vi "DataLog List Tag Logs.vi"(7 "database path":path, 11 "error in (no error)":errorcluster) -> (8 "tag info list":T1[](array[typedef]) {"logging parameters" format="%.2e"; "precision" items=["0", "1", "2", "3", "4", "5", "6", "7", "8", "9", "10", "11", "12", "13", "14", "15", "16", "17"]; "limit delay" format="%.2e"; "deadband" format="%.2e"}, 15 "error out":errorcluster)   [LabVIEW 2012]
doc: "List the tag log directories in the data log base path as well as any meta tag log directories contained in these. The validity of the logs will be verified and the tag infos will be loaded and returned in an array."
uses:
  typedefs/clusters/t_DataLog Tag Config.ctl
  typedefs/t_DataLog Temporal Types.ctl
  typedefs/t_DataLog Value Types.ctl
  typedefs/t_DataLog Numerical Format.ctl
  typedefs/t_DataLog Logging Algorithms.ctl
  typedefs/et_DataLog Meta Tag Specifier.ctl
  glb_DataLog MCVD.vi
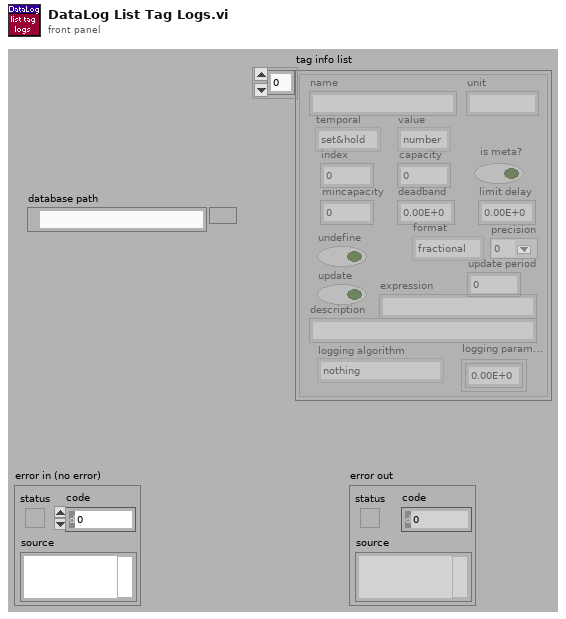
[diagram p1: front panel]
types:
  T1 = typedef "t_DataLog Tag Config.ctl" = cluster{"name":string, "unit":string, "temporal":T2, "value":T3, "index":i32, "capacity":i32, "is meta?":bool, "mincapacity":i32, "deadband":dbl, "limit delay":dbl, "format":T4, "precision":u8, "undefine":bool, "update":bool, "update period":u16, "expression":string, "description":string, "logging algorithm":T5, "logging parameters":dbl[]}
  T2 = typedef "t_DataLog Temporal Types.ctl" = enum16{"set&hold", "sample", "event"}
  T3 = typedef "t_DataLog Value Types.ctl" = enum16{"number", "string"}
  T4 = typedef "t_DataLog Numerical Format.ctl" = enum8{"fractional", "exponential", "engineering"}
  T5 = typedef "t_DataLog Logging Algorithms.ctl" = enum16{"nothing", "changes", "everything", "every Nth", "time threshold", "value threshold + prior", "t or v threshold", "t or v threshold + prior"}
  T6 = typedef "et_DataLog Meta Tag Specifier.ctl" = enum32{"warn_lo", "warn_hi", "A_lo", "A_hi", "B_lo", "B_hi", "C_lo", "C_hi", "D_lo", "D_hi", "E_lo", "E_hi", "F_lo", "F_hi", "G_lo", "G_hi", "H_lo", "H_hi", "I_lo", "I_hi", "J_lo", "J_hi", "K_lo", "K_hi", "L_lo", "L_hi", "M_lo", "M_hi", "N_lo", "N_hi", "min", "max", "not a meta"}
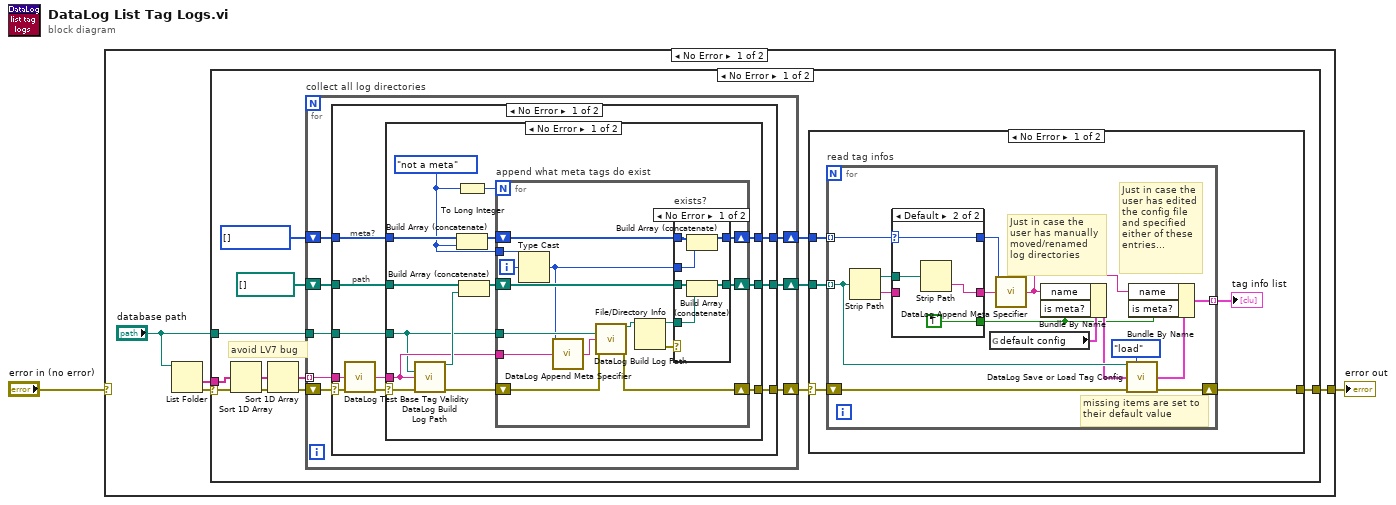
[diagram p0: block diagram]
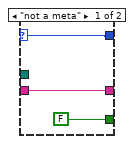
[diagram p2: hidden frame]
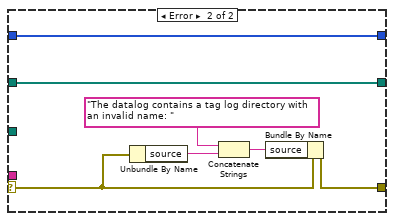
[diagram p5: hidden frame]
diagram:
  n1 = case shown="No Error" "error in (no error)" {
    selector: "error in (no error)" -> [_ w112]
    tunnel: [w6 w112] -> w2
    frame No Error {
      n2 = List Folder(path="database path") -> (folder names=w4:string[], error out=w5:errorcluster)  [unwired: 3 in, 2 out]
      n3 = case shown="No Error" w5 {
        selector: w5 -> [w16 w111]
        tunnel: [w14 w111] -> w6
        tunnel: w4 -> [w7 _]
        tunnel: "database path" -> [w10 _]
        frame No Error {
          w12 = T6[] [] items=["warn_lo", "warn_hi", "A_lo", "A_hi", "B_lo", "B_hi", "C_lo", "C_hi", "D_lo", "D_hi", "E_lo", "E_hi", "F_lo", "F_hi", "G_lo", "G_hi", "H_lo", "H_hi", "I_lo", "I_hi", "J_lo", "J_hi", "K_lo", "K_hi", "L_lo", "L_hi", "M_lo", "M_hi", "N_lo", "N_hi", "min", "max", "not a meta"]
          # "avoid LV7 bug"
          n4 = Sort 1D Array(array=w7) -> (sorted array=w9:string[])
          n5 = Sort 1D Array(array=w9) -> (sorted array=w8:string[])
          n6 = for "collect all log directories" {
            tunnel: w8 -> [w53] mode=indexing
            shift-right: [w49] -> w13
            shift-left: path[] [] -> [w50]
            shift-right: [w51] -> w15
            shift-left: w16 -> [w52]
            shift-right: [w47] -> w11
            shift-left: w12 -> [w48]
            tunnel: w10 -> [w46]
            n7 = case shown="No Error" w52 {
              selector: w52 -> [w62 w110]
              tunnel: w53 -> [w63 _]
              tunnel: [w60 w110] -> w51
              tunnel: w50 -> [w58 w109]
              tunnel: [w57 w109] -> w49
              tunnel: w48 -> [w56 w108]
              tunnel: [w55 w108] -> w47
              tunnel: w46 -> [w54 _]
              frame No Error {
                # "path"
                # "meta?"
                n8 = call "DataLog Test Base Tag Validity.vi"("base tag"=w63, "error in (no error)"=w62) -> ("base tag dup"=w59:string, "error out"=w61:errorcluster)  [unwired: 12 in]
                n9 = case shown="No Error" w61 {
                  selector: w61 -> [w77 w107]
                  tunnel: [w69 w106] -> w60
                  tunnel: w59 -> [w71 _]
                  tunnel: w58 -> [w76 w102]
                  tunnel: [w72 w102] -> w57
                  tunnel: w56 -> [w67 w101]
                  tunnel: [w66 w101] -> w55
                  tunnel: w54 -> [w64 _]
                  frame No Error {
                    w65 = et_DataLog_Meta_Tag_Specifier."not a meta" ("meta specifier (not a meta)")
                    n10 = call "DataLog Build Log Path.vi"("database path"=w64, "tag"=w71, "error in (no error)"=w77) -> ("tag log directory"=w75:path, "error out"=w70:errorcluster)  [unwired: 11 in]
                    n11 = To Long Integer(number=w65) -> (32bit integer=w74:i32)
                    n12 = Build Array (concatenate)(w67, w65) -> (w68:T6[])
                    n13 = Build Array (concatenate)(w76, w75) -> (w73:path[])
                    n14 = for "append what meta tags do exist" {
                      N: w74 -> [_]
                      shift-right: [w85] -> w72
                      shift-left: w73 -> [w86]
                      tunnel: w71 -> [w80]
                      tunnel: w65 -> [w91]
                      shift-right: [w89] -> w69
                      shift-left: w70 -> [w90]
                      shift-right: [w83] -> w66
                      shift-left: w68 -> [w82]
                      tunnel: w64 -> [w81]
                      i -> [w92]
                      n15 = Type Cast(type=w91, x=w92) -> (*(type *) &x=w78:T6)
                      n16 = call "DataLog Append Meta Specifier.vi"("meta specifier"=w78, "tag in"=w80) -> ("tag out"=w79:string)  [unwired: 13 in]
                      n17 = call "DataLog Build Log Path.vi"("database path"=w81, "tag"=w79, "error in (no error)"=w90) -> ("tag log directory"=w88:path, "error out"=w89:errorcluster)  [unwired: 11 in]
                      n18 = File/Directory Info(path=w88) -> (path out=w84:path, error out=w87:errorcluster)  [unwired: 1 in, 5 out]
                      n19 = case "exists?" shown="No Error" w87 {
                        tunnel: w86 -> [w98 w100]
                        tunnel: [w97 w100] -> w85
                        tunnel: w84 -> [w96 _]
                        tunnel: w82 -> [w95 w99]
                        tunnel: [w94 w99] -> w83
                        tunnel: w78 -> [w93 _]
                        frame No Error {
                          n20 = Build Array (concatenate)(w95, w93) -> (w94:T6[])
                          n21 = Build Array (concatenate)(w98, w96) -> (w97:path[])
                        }
                        frame Error {
                        }
                      }
                    }
                  }
                  frame Error {
                    n22 = Unbundle By Name(w107) -> ("source"=w105:string)
                    n23 = Concatenate Strings("The datalog contains a tag log directory with an invalid name: " ("string"), w105) -> (w103:string)
                    n24 = Bundle By Name(cluster=w107, "source"=w103) -> (w106:errorcluster)
                  }
                }
              }
              frame Error {
              }
            }
          }
          n25 = case shown="No Error" w15 {
            selector: w15 -> [w21 w45]
            tunnel: [w20 w45] -> w14
            tunnel: w13 -> [w22 _]
            tunnel: w11 -> [w18 _]
            frame No Error {
              n26 = for "read tag infos" {
                tunnel: w22 -> [w32] mode=indexing
                shift-right: [w30] -> w20
                shift-left: w21 -> [w31]
                tunnel: [w25] -> w19 mode=indexing
                tunnel: w18 -> [w37] mode=indexing
                # "Just in case the\nuser has edited\nthe config file\nand specified\neither of these\nentries..."
                # "Just in case the\nuser has manually\nmoved/renamed\nlog directories"
                # "missing items are set to\ntheir default value"
                n27 = Strip Path(path=w32) -> (stripped path=w36:path, name=w35:string)
                n28 = case shown="Default" w37 {
                  selector: w37 -> [w39 w42]
                  tunnel: w36 -> [_ w44]
                  tunnel: [w40 w43] -> w33
                  tunnel: w35 -> [w40 _]
                  tunnel: [w39 w42] -> w34
                  tunnel: [FALSE TRUE] -> w23
                  frame "not a meta" {
                  }
                  frame Default {
                    n29 = Strip Path(path=w44) -> (name=w43:string)  [unwired: 1 out]
                  }
                }
                n30 = global read "glb_DataLog MCVD.vi" "default config"() -> (w28:T1)
                n31 = call "DataLog Append Meta Specifier.vi"("meta specifier"=w34, "tag in"=w33) -> ("tag out"=w24:string)  [unwired: 13 in]
                n32 = Bundle By Name(cluster=w28, "name"=w24, "is meta?"=w23) -> (w27:T1)
                n33 = call "DataLog Save or Load Tag Config.vi"("tag log directory"=w32, "action"=enum16{"save", "load"}."load", "tag config in"=w27, "error in (no error)"=w31) -> ("tag config out"=w26:T1, "error out"=w30:errorcluster)  [unwired: 9 in, 1 out]
                n34 = Bundle By Name(cluster=w26, "name"=w24, "is meta?"=w23) -> (w25:T1)
              }
              "tag info list" <- w19
            }
            frame Error {
            }
          }
        }
        frame Error {
        }
      }
    }
    frame Error {
    }
  }
  "error out" <- w2
